vi "LoopselFF_2cam_continouos.VI"() -> ()   [LabVIEW 2015]
panel:
  in  "start continouos":bool
  out "cams recognised":u8=2
  in  "cam select\n1: cam 1\n2: cam 2\n3: both cams":u8=3
  out "Signalverlaufgraph 2":u16[](graph)=[542, 542, 543, 543, 0, 1, 0, 468, 2, 2, 3, 3, 4, 4, 5, 5, 6, 6, 7, 7, 8, 8, 9, 9, 10, 10, 11, 11, 12, 12, 13, 13, 14, 14, 15, 15, 16, 16, 17, 17, 18, 18, 19, 19, 20, 20, 21, 21, 22, 22, 23, 23, 24, 24, 25, 25, 26, 26, 27, 27, 28, 28, 29, 29, 30, 30, 31, 31, 32, 32, 33, 33, 34, 34, 35, 35, 36, 36, 37, 37, 38, 38, 39, 39, 40, 40, 41, 41, 42, 42, 43, 43, 44, 44, 45, 45, 46, 46, 47, 47, 48, 48, 49, 49, 50, 50, 51, 51, 52, 52, 53, 53, 54, 54, 55, 55, 56, 56, 57, 57, 58, 58, 59, 59, 60, 60, 61, 61, 62, 62, 63, 63, 64, 64, 65, 65, 66, 66, 67, 67, 68, 68, 69, 69, 70, 70, 71, 71, 72, 72, 73, 73, 74, 74, 75, 75, 76, 76, 77, 77, 78, 78, 79, 79, 80, 80, 81, 81, 82, 82, 83, 83, 84, 84, 85, 85, 86, 86, 87, 87, 88, 88, 89, 89, 90, 90, 91, 91, 92, 92, 93, 93, 94, 94, 95, 95, 96, 96, 97, 97, 98, 98, 99, 99, 100, 100, 101, 101, 102, 102, 103, 103, 104, 104, 105, 105, 106, 106, 107, 107, 108, 108, 109, 109, 110, 110, 111, 111, 112, 112, 113, 113, 114, 114, 115, 115, 116, 116, 117, 117, 118, 118, 119, 119, 120, 120, 121, 121, 122, 122, 123, 123, 124, 124, 125, 125, 126, 126, 127, 127, 128, 128, 129, 129, 130, 130, 131, 131, 132, 132, 133, 133, 134, 134, 135, 135, 136, 136, 137, 137, 138, 138, 139, 139, 140, 140, 141, 141, 142, 142, 143, 143, 144, 144, 145, 145, 146, 146, 147, 147, 148, 148, 149, 149, 150, 150, 151, 151, 152, 152, 153, 153, 154, 154, 155, 155, 156, 156, 157, 157, 158, 158, 159, 159, 160, 160, 161, 161, 162, 162, 163, 163, 164, 164, 165, 165, 166, 166, 167, 167, 168, 168, 169, 169, 170, 170, 171, 171, 172, 172, 173, 173, 174, 174, 175, 175, 176, 176, 177, 177, 178, 178, 179, 179, 180, 180, 181, 181, 182, 182, 183, 183, 184, 184, 185, 185, 186, 186, 187, 187, 188, 188, 189, 189, 190, 190, 191, 191, 192, 192, 193, 193, 194, 194, 195, 195, 196, 196, 197, 197, 198, 198, 199, 199, 200, 200, 201, 201, 202, 202, 203, 203, 204, 204, 205, 205, 206, 206, 207, 207, 208, 208, 209, 209, 210, 210, 211, 211, 212, 212, 213, 213, 214, 214, 215, 215, 216, 216, 217, 217, 218, 218, 219, 219, 220, 220, 221, 221, 222, 222, 223, 223, 224, 224, 225, 225, 226, 226, 227, 227, 228, 228, 229, 229, 230, 230, 231, 231, 232, 232, 233, 233, 234, 234, 235, 235, 236, 236, 237, 237, 238, 238, 239, 239, 240, 240, 241, 241, 242, 242, 243, 243, 244, 244, 245, 245, 246, 246, 247, 247, 248, 248, 249, 249, 250, 250, 251, 251, 252, 252, 253, 253, 254, 254, 255, 255, 256, 256, 257, 257, 258, 258, 259, 259, 260, 260, 261, 261, 262, 262, 263, 263, 264, 264, 265, 265, 266, 266, 267, 267, 268, 268, 269, 269, 270, 270, 271, 271, 272, 272, 273, 273, 274, 274, 275, 275, 276, 276, 277, 277, 278, 278, 279, 279, 280, 280, 281, 281, 282, 282, 283, 283, 284, 284, 285, 285, 286, 286, 287, 287, 288, 288, 289, 289, 290, 290, 291, 291, 292, 292, 293, 293, 294, 294, 295, 295, 296, 296, 297, 297, 298, 298, 299, 299, 300, 300, 301, 301, 302, 302, 303, 303, 304, 304, 305, 305, 306, 306, 307, 307, 308, 308, 309, 309, 310, 310, 311, 311, 312, 312, 313, 313, 314, 314, 315, 315, 316, 316, 317, 317, 318, 318, 319, 319, 320, 320, 321, 321, 322, 322, 323, 323, 324, 324, 325, 325, 326, 326, 327, 327, 328, 328, 329, 329, 330, 330, 331, 331, 332, 332, 333, 333, 334, 334, 335, 335, 336, 336, 337, 337, 338, 338, 339, 339, 340, 340, 341, 341, 342, 342, 343, 343, 344, 344, 345, 345, 346, 346, 347, 347, 348, 348, 349, 349, 350, 350, 351, 351, 352, 352, 353, 353, 354, 354, 355, 355, 356, 356, 357, 357, 358, 358, 359, 359, 360, 360, 361, 361, 362, 362, 363, 363, 364, 364, 365, 365, 366, 366, 367, 367, 368, 368, 369, 369, 370, 370, 371, 371, 372, 372, 373, 373, 374, 374, 375, 375, 376, 376, 377, 377, 378, 378, 379, 379, 380, 380, 381, 381, 382, 382, 383, 383, 384, 384, 385, 385, 386, 386, 387, 387, 388, 388, 389, 389, 390, 390, 391, 391, 392, 392, 393, 393, 394, 394, 395, 395, 396, 396, 397, 397, 398, 398, 399, 399, 400, 400, 401, 401, 402, 402, 403, 403, 404, 404, 405, 405, 406, 406, 407, 407, 408, 408, 409, 409, 410, 410, 411, 411, 412, 412, 413, 413, 414, 414, 415, 415, 416, 416, 417, 417, 418, 418, 419, 419, 420, 420, 421, 421, 422, 422, 423, 423, 424, 424, 425, 425, 426, 426, 427, 427, 428, 428, 429, 429, 430, 430, 431, 431, 432, 432, 433, 433, 434, 434, 435, 435, 436, 436, 437, 437, 438, 438, 439, 439, 440, 440, 441, 441, 442, 442, 443, 443, 444, 444, 445, 445, 446, 446, 447, 447, 448, 448, 449, 449, 450, 450, 451, 451, 452, 452, 453, 453, 454, 454, 455, 455, 456, 456, 457, 457, 458, 458, 459, 459, 460, 460, 461, 461, 462, 462, 463, 463, 464, 464, 465, 465, 466, 466, 467, 467, 468, 468, 469, 469, 470, 470, 471, 471, 472, 472, 473, 473, 474, 474, 475, 475, 476, 476, 477, 477, 478, 478, 479, 479, 480, 480, 481, 481, 482, 482, 483, 483, 484, 484, 485, 485, 486, 486, 487, 487, 488, 488, 489, 489, 490, 490, 491, 491, 492, 492, 493, 493, 494, 494, 495, 495, 496, 496, 497, 497, 498, 498, 499, 499, 500, 500, 501, 501, 502, 502, 503, 503, 504, 504, 505, 505, 506, 506, 507, 507, 508, 508, 509, 509, 510, 510, 511, 511, 512, 512, 513, 513, 514, 514, 515, 515, 516, 516, 517, 517, 518, 518, 519, 519, 520, 520, 521, 521, 522, 522, 523, 523, 524, 524, 525, 525, 526, 526, 527, 527, 528, 528, 529, 529, 530, 530, 531, 531, 532, 532, 533, 533, 534, 534, 535, 535, 536, 536, 537, 537, 538, 538, 539, 539, 540, 540, 541, 541]
  out "FIFO overflow 2":bool
  in  "alloc mem":bool
  out "FREE \nRAM MB":u64=14868
  out "BUILT-IN\nRAM MB":u64=18530
  out "SEC":dbl=0.02
  out "MB RAM":u64=2
  in  "pos slope":u8=1
  in  "both slopes":u8
  in  "DAT in 10ns":u32
  out "FIFO overflow":bool
  in  "extTrig 0/1":u8
  in  "stop all":bool
  in  "Slide":u32(slide)=469 scale=1.0..1000.0
  in  "frequency[Hz]":u32
  in  "no.of samples (nos)":u32=1000
  in  "exposuretime[ms]":dbl=0.02 format="%.3f"
  out "Signalverlaufgraph":u16[](graph)=[0, 0, 0, 0, 0, 1, 0, 468, 0, 0, 0, 0, 0, 0, 0, 0, 0, 0, 0, 0, 0, 0, 0, 0, 0, 0, 0, 0, 0, 0, 0, 0, 0, 0, 0, 0, 0, 0, 0, 0, 0, 0, 0, 0, 0, 0, 0, 0, 0, 0, 0, 0, 0, 0, 0, 0, 0, 0, 0, 0, 0, 0, 0, 0, 0, 0, 0, 0, 0, 0, 0, 0, 0, 0, 0, 0, 0, 0, 0, 0, 0, 0, 0, 0, 0, 0, 0, 0, 0, 0, 0, 0, 0, 0, 0, 0, 0, 0, 0, 0, 0, 0, 0, 0, 0, 0, 0, 0, 0, 0, 0, 0, 0, 0, 0, 0, 0, 0, 0, 0, 0, 0, 0, 0, 0, 0, 0, 0, 0, 0, 0, 0, 0, 0, 0, 0, 0, 0, 0, 0, 0, 0, 0, 0, 0, 0, 0, 0, 0, 0, 0, 0, 0, 0, 0, 0, 0, 0, 0, 0, 0, 0, 0, 0, 0, 0, 0, 0, 0, 0, 0, 0, 0, 0, 0, 0, 0, 0, 0, 0, 0, 0, 0, 0, 0, 0, 0, 0, 0, 0, 0, 0, 0, 0, 0, 0, 0, 0, 0, 0, 0, 0, 0, 0, 0, 0, 0, 0, 0, 0, 0, 0, 0, 0, 0, 0, 0, 0, 0, 0, 0, 0, 0, 0, 0, 0, 0, 0, 0, 0, 0, 0, 0, 0, 0, 0, 0, 0, 0, 0, 0, 0, 0, 0, 0, 0, 0, 0, 0, 0, 0, 0, 0, 0, 0, 0, 0, 0, 0, 0, 0, 0, 0, 0, 0, 0, 0, 0, 0, 0, 0, 0, 0, 0, 0, 0, 0, 0, 0, 0, 0, 0, 0, 0, 0, 0, 0, 0, 0, 0, 0, 0, 0, 0, 0, 0, 0, 0, 0, 0, 0, 0, 0, 0, 0, 0, 0, 0, 0, 0, 0, 0, 0, 0, 0, 0, 0, 0, 0, 0, 0, 0, 0, 0, 0, 0, 0, 0, 0, 0, 0, 0, 0, 0, 0, 0, 0, 0, 0, 0, 0, 0, 0, 0, 0, 0, 0, 0, 0, 0, 0, 0, 0, 0, 0, 0, 0, 0, 0, 0, 0, 0, 0, 0, 0, 0, 0, 0, 0, 0, 0, 0, 0, 0, 0, 0, 0, 0, 0, 0, 0, 0, 0, 0, 0, 0, 0, 0, 0, 0, 0, 0, 0, 0, 0, 0, 0, 0, 0, 0, 0, 0, 0, 0, 0, 0, 0, 0, 0, 0, 0, 0, 0, 0, 0, 0, 0, 0, 0, 0, 0, 0, 0, 0, 0, 0, 0, 0, 0, 0, 0, 0, 0, 0, 0, 0, 0, 0, 0, 0, 0, 0, 0, 0, 0, 0, 0, 0, 0, 0, 0, 0, 0, 0, 0, 0, 0, 0, 0, 0, 0, 0, 0, 0, 0, 0, 0, 0, 0, 0, 0, 0, 0, 0, 0, 0, 0, 0, 0, 0, 0, 0, 0, 0, 0, 0, 0, 0, 0, 0, 0, 0, 0, 0, 0, 0, 0, 0, 0, 0, 0, 0, 0, 0, 0, 0, 0, 0, 0, 0, 0, 0, 0, 0, 0, 0, 0, 0, 0, 0, 0, 0, 0, 0, 0, 0, 0, 0, 0, 0, 0, 0, 0, 0, 0, 0, 0, 0, 0, 0, 0, 0, 0, 0, 0, 0, 0, 0, 0, 0, 0, 0, 0, 0, 0, 0, 0, 0, 0, 0, 0, 0, 0, 0, 0, 0, 0, 0, 0, 0, 0, 0, 0, 0, 0, 0, 0, 0, 0, 0, 0, 0, 0, 0, 0, 0, 0, 0, 0, 0, 0, 0, 0, 0, 0, 0, 0, 0, 0, 0, 0, 0, 0, 0, 0, 0, 0, 0, 0, 0, 0, 0, 0, 0, 0, 0, 0, 0, 0, 0, 0, 0, 0, 0, 0, 0, 0, 0, 0, 0, 0, 0, 0, 0, 0, 0, 0, 0, 0, 0, 0, 0, 0, 0, 0, 0, 0, 0, 0, 0, 0, 0, 0, 0, 0, 0, 0, 0, 0, 0, 0, 0, 0, 0, 0, 0, 0, 0, 0, 0, 0, 0, 0, 0, 0, 0, 0, 0, 0, 0, 0, 0, 0, 0, 0, 0, 0, 0, 0, 0, 0, 0, 0, 0, 0, 0, 0, 0, 0, 0, 0, 0, 0, 0, 0, 0, 0, 0, 0, 0, 0, 0, 0, 0, 0, 0, 0, 0, 0, 0, 0, 0, 0, 0, 0, 0, 0, 0, 0, 0, 0, 0, 0, 0, 0, 0, 0, 0, 0, 0, 0, 0, 0, 0, 0, 0, 0, 0, 0, 0, 0, 0, 0, 0, 0, 0, 0, 0, 0, 0, 0, 0, 0, 0, 0, 0, 0, 0, 0, 0, 0, 0, 0, 0, 0, 0, 0, 0, 0, 0, 0, 0, 0, 0, 0, 0, 0, 0, 0, 0, 0, 0, 0, 0, 0, 0, 0, 0, 0, 0, 0, 0, 0, 0, 0, 0, 0, 0, 0, 0, 0, 0, 0, 0, 0, 0, 0, 0, 0, 0, 0, 0, 0, 0, 0, 0, 0, 0, 0, 0, 0, 0, 0, 0, 0, 0, 0, 0, 0, 0, 0, 0, 0, 0, 0, 0, 0, 0, 0, 0, 0, 0, 0, 0, 0, 0, 0, 0, 0, 0, 0, 0, 0, 0, 0, 0, 0, 0, 0, 0, 0, 0, 0, 0, 0, 0, 0, 0, 0, 0, 0, 0, 0, 0, 0, 0, 0, 0, 0, 0, 0, 0, 0, 0, 0, 0, 0, 0, 0, 0, 0, 0, 0, 0, 0, 0, 0, 0, 0, 0, 0, 0, 0, 0, 0, 0, 0, 0, 0, 0, 0, 0, 0, 0, 0, 0, 0, 0, 0, 0, 0, 0, 0, 0, 0, 0, 0, 0, 0, 0, 0, 0, 0, 0, 0, 0, 0, 0, 0, 0, 0, 0, 0, 0, 0, 0, 0, 0, 0, 0, 0, 0, 0, 0, 0, 0, 0, 0, 0, 0, 0, 0, 0, 0, 0, 0, 0, 0, 0, 0, 0, 0, 0, 0, 0, 0, 0, 0, 0, 0, 0, 0, 0, 0, 0, 0, 0, 0, 0, 0, 0, 0, 0, 0, 0, 0, 0, 0, 0, 0, 0, 0, 0, 0, 0, 0, 0, 0, 0, 0, 0, 0, 0, 0, 0, 0, 0, 0, 0, 0, 0, 0, 0, 0, 0, 0, 0, 0, 0, 0, 0, 0, 0, 0, 0, 0, 0, 0, 0, 0, 0, 0, 0, 0, 0, 0, 0, 0, 0, 0, 0, 0, 0, 0, 0, 0, 0, 0, 0, 0, 0, 0, 0, 0, 0, 0, 0, 0, 0, 0, 0, 0, 0, 0, 0, 0, 0, 0]
  # "Start with run"
  # "Abort with ESC"
  # "press Esc to stop measurement"
  # "1x"
  # "exit here"
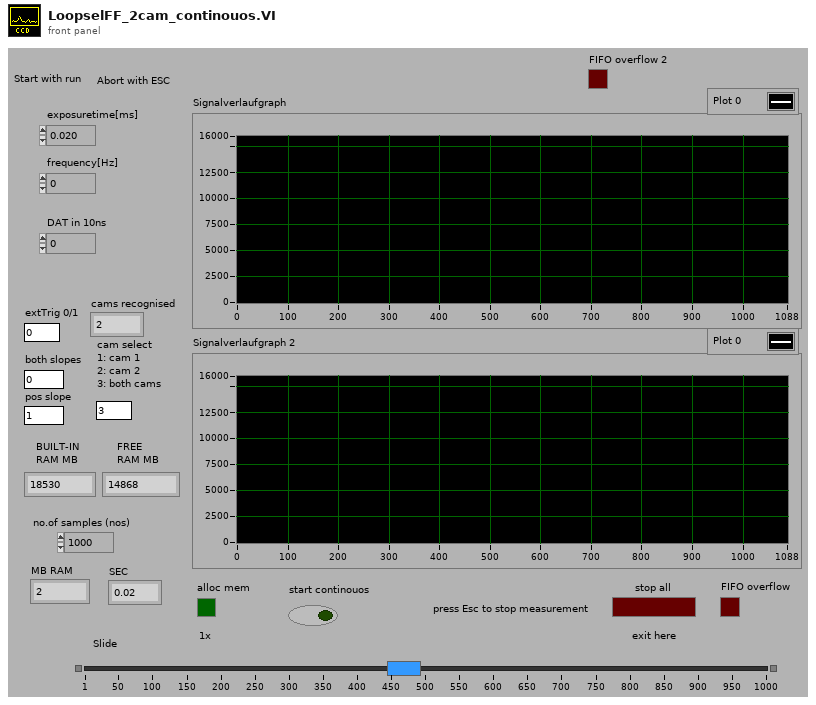
[diagram p1: front panel]
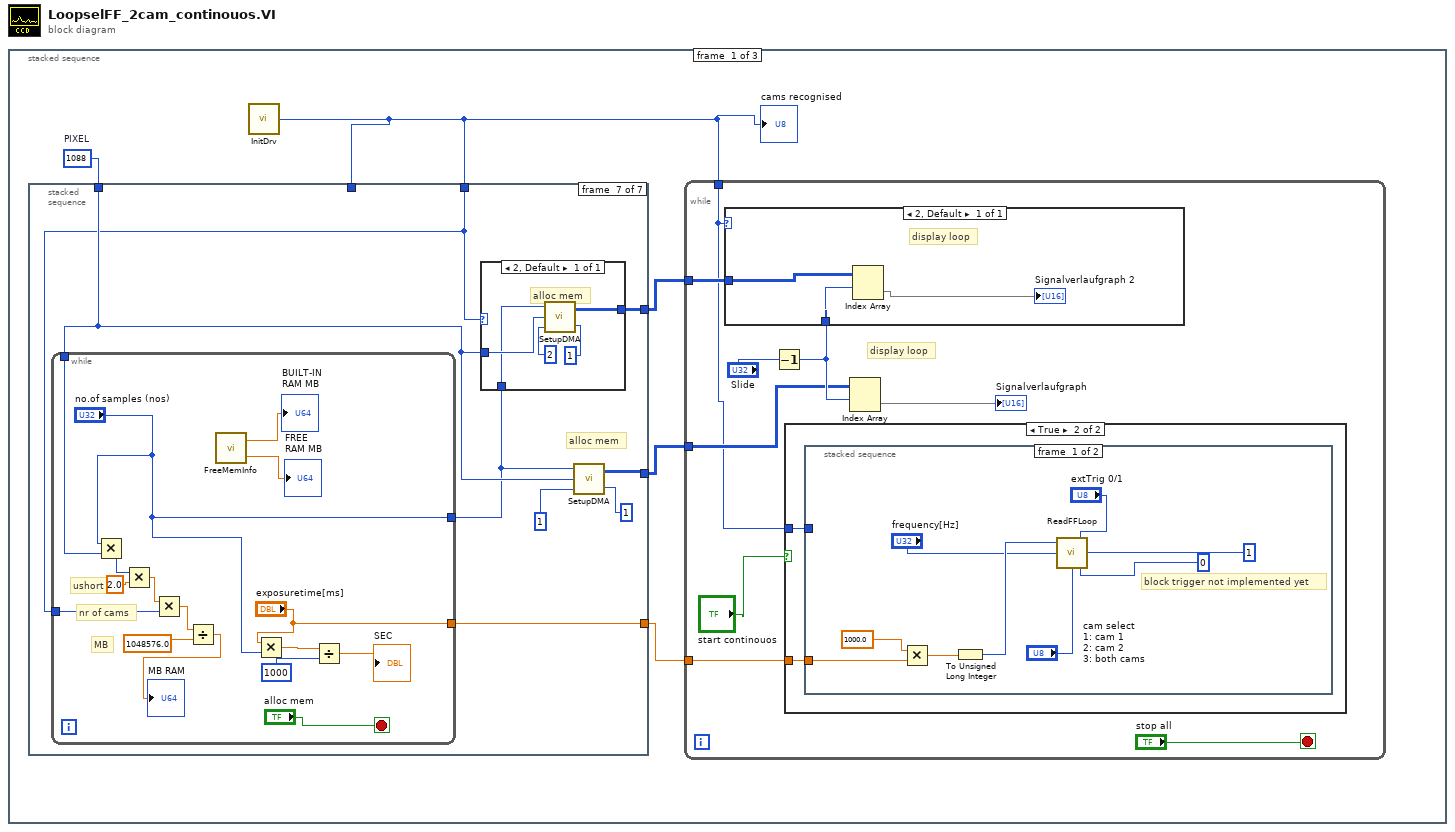
[diagram p0: block diagram]
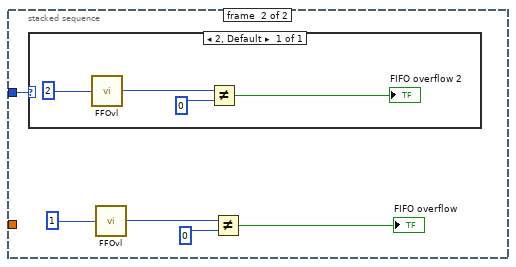
[diagram p3: hidden frame]
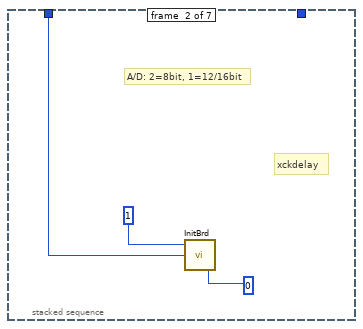
[diagram p5: hidden frame]
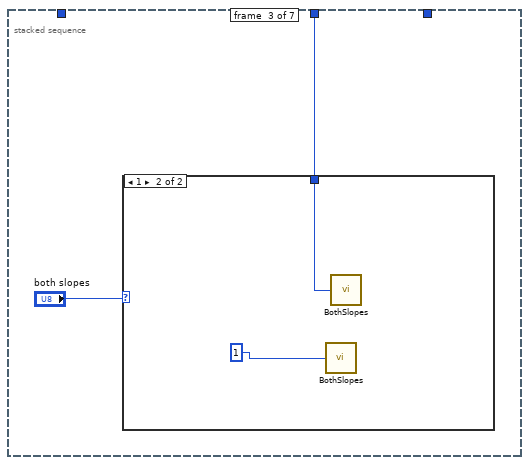
[diagram p6: hidden frame]
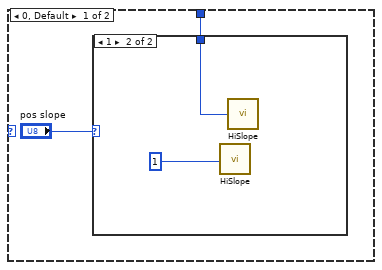
[diagram p7: hidden frame]
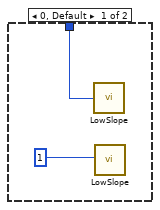
[diagram p8: hidden frame]
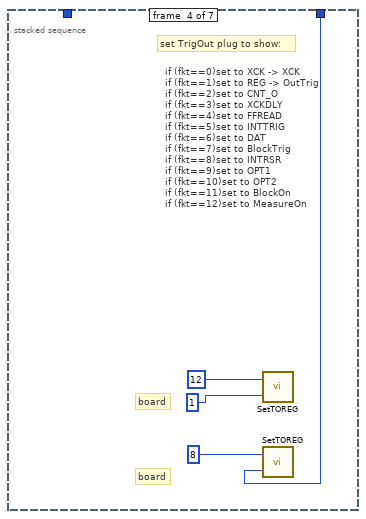
[diagram p9: hidden frame]
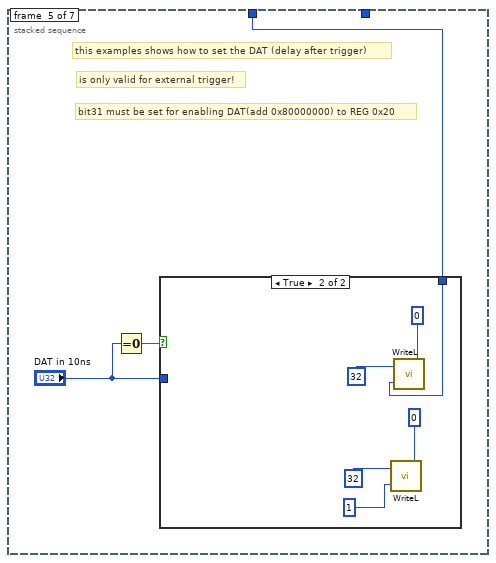
[diagram p10: hidden frame]
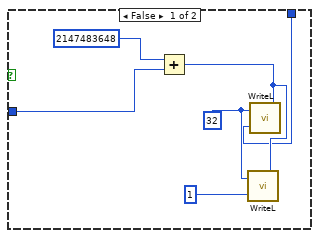
[diagram p11: hidden frame]
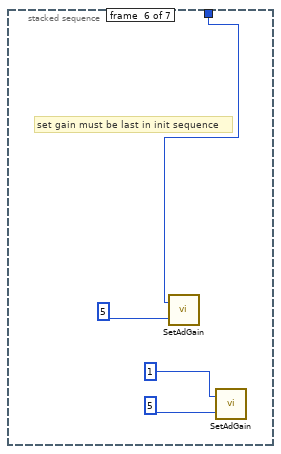
[diagram p12: hidden frame]
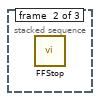
[diagram p13: hidden frame]
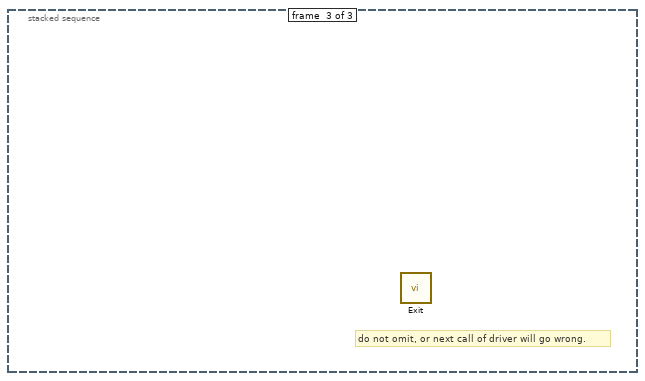
[diagram p14: hidden frame]
diagram:
  n1 = stacked-sequence {
    frame #0 {
      w5 = u32 1088  # PIXEL
      n2 = call "InitDrv.vi"() -> ("Boards"=w1:u8)  [unwired: 1 in]
      "cams recognised" <- w1
      n3 = stacked-sequence {
        tunnel: [_ _ _ _ _ _ w80] -> w2
        tunnel: w5 -> [_ w38 _ _ _ _ w78]
        tunnel: w1 -> [_ _ _ _ _ _ w74]
        tunnel: [_ _ _ _ _ _ w76] -> w4
        tunnel: [_ _ _ _ _ _ w75] -> w3
        tunnel: w1 -> [_ _ w41 w51 w55 w70 _]
        frame #0 {
        }
        frame #1 {
          # "xckdelay"
          # "A/D: 2=8bit, 1=12/16bit"
          n4 = call "InitBrd.vi"("xckdly"=u32 0, "pixel"=w38, "flag816"=u32 1) -> ()  [unwired: 3 in]
        }
        frame #2 {
          n5 = case shown="1" "both slopes" {
            tunnel: w41 -> [w43 w50]
            frame 0, Default {
              n6 = case shown="1" "pos slope" {
                tunnel: w43 -> [w46 w48]
                frame 0, Default {
                  n7 = call "LowSlope.vi"("board"=w46) -> ()  [unwired: 1 in]
                  n8 = call "LowSlope.vi"("board"=1) -> ()  [unwired: 1 in]
                }
                frame 1 {
                  n9 = call "HiSlope.vi"("board"=1) -> ()  [unwired: 1 in]
                  n10 = call "HiSlope.vi"("board"=w48) -> ()  [unwired: 1 in]
                }
              }
            }
            frame 1 {
              n11 = call "BothSlopes.vi"("board"=1) -> ()  [unwired: 1 in]
              n12 = call "BothSlopes.vi"("board"=w50) -> ()  [unwired: 1 in]
            }
          }
        }
        frame #3 {
          # "board"
          # "board"
          # "set TrigOut plug to show:"
          # "if (fkt==0)set to XCK -> XCK\nif (fkt==1)set to REG -> OutTrig\nif (fkt==2)set to CNT_O\nif (fkt==3)set to XCKDLY\nif (fkt==4)set to FFREAD\nif (fkt==5)set to INTTRIG\nif (fkt==6)set to DAT\nif (fkt==7)set to BlockTrig\nif (fkt==8)set to INTRSR\nif (fkt==9)set to OPT1\nif (fkt==10)set to OPT2\nif (fkt==11)set to BlockOn\nif (fkt==12)set to MeasureOn"
          n13 = call "SetTOREG.vi"("board"=u8 1, "fkt"=u8 12) -> ()  [unwired: 1 in]
          n14 = call "SetTOREG.vi"("board"=w51, "fkt"=u8 8) -> ()  [unwired: 1 in]
        }
        frame #4 {
          # "bit31 must be set for enabling DAT(add 0x80000000) to REG 0x20"
          # "is only valid for external trigger!"
          # "this examples shows how to set the DAT (delay after trigger)"
          n15 = Equal To 0?(x="DAT in 10ns") -> (x = 0?=w57:bool)
          n16 = case shown="True" w57 {
            tunnel: "DAT in 10ns" -> [w62 _]
            tunnel: w55 -> [w59 w67]
            frame False {
              w61 = u32 32
              n17 = Add(x=u32 2147483648, y=w62) -> (x+y=w60:u32)
              n18 = call "WriteL.vi"("val"=w60, "board"=1, "offset"=w61) -> ()
              n19 = call "WriteL.vi"("val"=w60, "board"=w59, "offset"=w61) -> ()
            }
            frame True {
              n20 = call "WriteL.vi"("val"=0, "board"=1, "offset"=u32 32) -> ()
              n21 = call "WriteL.vi"("val"=0, "board"=w67, "offset"=u32 32) -> ()
            }
          }
        }
        frame #5 {
          # "set gain must be last in init sequence"
          n22 = call "SetAdGain.vi"("gain"=u8 5, "board"=w70) -> ()  [unwired: 1 in]
          n23 = call "SetAdGain.vi"("gain"=u8 5, "board"=u8 1) -> ()  [unwired: 1 in]
        }
        frame #6 {
          # "alloc mem"
          n24 = while {
            tunnel: w78 -> [w88]
            tunnel: ["exposuretime[ms]"] -> w80
            tunnel: ["no.of samples (nos)"] -> w77
            tunnel: w74 -> [w87]
            stop <- "alloc mem" stop-if-true
            # "nr of cams"
            # "MB"
            # "ushort"
            n25 = Multiply(x="no.of samples (nos)", y=w88) -> (x*y=w93:u32)
            n26 = Multiply(x=w93, y=2.0) -> (x*y=w94:dbl)
            n27 = Multiply(x=w94, y=w87) -> (x*y=w95:dbl)
            n28 = Divide(x=w95, y=1048576.0) -> (x/y=→"MB RAM":dbl)
            n29 = call "FreeMemInfo.vi"() -> ("PhysicalSpace"=→"BUILT-IN\nRAM MB":dbl, "PhysicalFreeSpace"=→"FREE \nRAM MB":dbl)  [unwired: 1 in]
            n30 = Multiply(x="exposuretime[ms]", y="no.of samples (nos)") -> (x*y=w100:dbl)
            n31 = Divide(x=w100, y=1000) -> (x/y=→"SEC":dbl)
          }
          n32 = case shown="2, Default" w74 {
            tunnel: w78 -> [w84]
            tunnel: w77 -> [w83]
            tunnel: [w82] -> w76
            frame 2, Default {
              # "alloc mem"
              n33 = call "SetupDMA.vi"("blocks"=1, "Drv"=2, "pixel"=w84, "nos"=w83) -> ("Data Values"=w82:u16[][])
            }
          }
          n34 = call "SetupDMA.vi"("blocks"=1, "Drv"=1, "pixel"=w78, "nos"=w77) -> ("Data Values"=w75:u16[][])
        }
      }
      n35 = while {
        tunnel: w4 -> [w11]
        tunnel: w3 -> [w10]
        tunnel: w2 -> [w8]
        tunnel: w1 -> [w7]
        stop <- "stop all" stop-if-true
        # "display loop"
        n36 = Decrement(x="Slide") -> (x-1=w13:u32)
        n37 = case shown="2, Default" w7 {
          tunnel: w13 -> [w37]
          tunnel: w11 -> [w36]
          frame 2, Default {
            # "display loop"
            n38 = Index Array(array=w36, index (row)=w37) -> (element=→"Signalverlaufgraph 2":u16[])  [unwired: 1 in]
          }
        }
        n39 = case shown="True" "start continouos" {
          tunnel: w8 -> [_ w16]
          tunnel: w7 -> [_ w15]
          frame False {
          }
          frame True {
            n40 = stacked-sequence {
              tunnel: w16 -> [w18 _]
              tunnel: w15 -> [_ w26]
              frame #0 {
                # "block trigger not implemented yet"
                n41 = Multiply(x=1000.0, y=w18) -> (x*y=w20:dbl)
                n42 = To Unsigned Long Integer(number=w20) -> (unsigned 32bit integer=w25:u32)
                n43 = call "ReadFFLoop.vi"("blocktrigger"=u8 0, "btrig_ch"=u8 1, "ExtTrig"="extTrig 0/1", "cam_sel"="cam select\n1: cam 1\n2: cam 2\n3: both cams", "freq"="frequency[Hz]", "exptus"=w25) -> ()
              }
              frame #1 {
                n44 = case shown="2, Default" w26 {
                  frame 2, Default {
                    n45 = call "FFOvl.vi"("Drv"=2) -> ("FFOvl"=w32:u8)
                    n46 = Not Equal?(x=w32, y=0) -> (x != y?=→"FIFO overflow 2":bool)
                  }
                }
                n47 = call "FFOvl.vi"("Drv"=1) -> ("FFOvl"=w29:u8)
                n48 = Not Equal?(x=w29, y=0) -> (x != y?=→"FIFO overflow":bool)
              }
            }
          }
        }
        n49 = Index Array(array=w10, index (row)=w13) -> (element=→"Signalverlaufgraph":u16[])  [unwired: 1 in]
      }
    }
    frame #1 {
      n50 = call "FFStop.vi"() -> ()  [unwired: 1 in]
    }
    frame #2 {
      # "do not omit, or next call of driver will go wrong."
      n51 = call "Exit.vi"() -> ()  [unwired: 1 in]
    }
  }
